vi "Add_Source.vi"(5 "project":refnum<vi>, 7 "IB_Destination.lvclass":refnum<class "IB_Destination.lvclass">, 8 "error in (no error)":errorcluster, 9 "project items":refnum<class "IB_Tree_Item_Proj.lvclass">[](array[class]), 10 "source in":refnum<class "IB_Source.lvclass">[](array[class]), 11 "IB_DestTree in":refnum<class "IB_Tree_Dest.lvclass">) -> (0 "error out":errorcluster, 1 "updated project items":refnum<class "IB_Tree_Item_Proj.lvclass">[](array[class]), 2 "source out":refnum<class "IB_Source.lvclass">[](array[class]), 3 "IB_DestTree out":refnum<class "IB_Tree_Dest.lvclass">)   [LabVIEW 2020, in "IB_Tree_Dest.lvclass"]
uses:
  <vilib>/AppBuilder/IB_Classes/Tree_Dest/IB_Tree_Dest.lvclass
  <vilib>/AppBuilder/IB_Classes/Tree_Dest/IB_Tree_Dest.lvclass/IB_Tree_Dest.ctl
  <vilib>/AppBuilder/IB_Classes/Source/IB_Source.lvclass
  <vilib>/AppBuilder/IB_Classes/Tree/IB_Tree.lvclass
  <vilib>/AppBuilder/IB_Classes/Tree_Item_Proj/IB_Tree_Item_Proj.lvclass
  <vilib>/AppBuilder/IB_Classes/Destination/IB_Destination.lvclass
  <vilib>/AppBuilder/IB_Classes/Tree_Item_Source/IB_Tree_Item_Source.lvclass
  e:/builds/penguin/labview/branches/2020/dev/dist/vi.lib/AppBuilder/IB_Classes/Tree/IB_Tree.lvclass
  e:/builds/penguin/labview/branches/2020/dev/dist/vi.lib/AppBuilder/IB_Classes/Tree_Dest/IB_Tree_Dest.lvclass
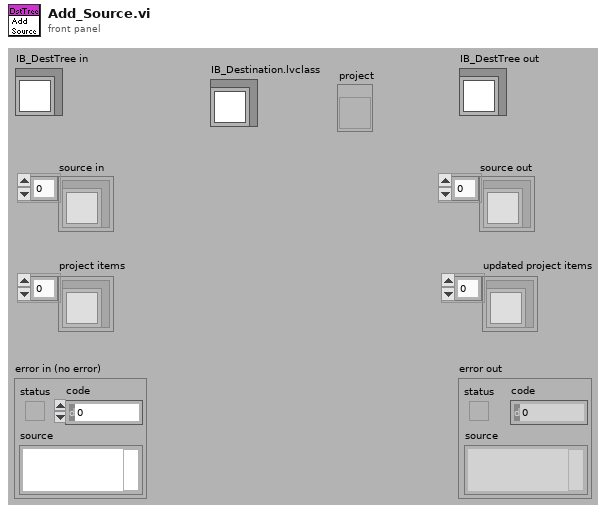
[diagram p1: front panel]
types:
  T1 = typedef "IB_Destination.ctl" = cluster{"name":string, "unlock":bool, "parentTag":string, "destTag":string, "eng_installPath":string}
  T2 = typedef "IB_Tree_Item_Proj.ctl" = cluster{"itemID":string, "path":path}
  T3 = typedef "IB_Source.ctl" = cluster{"name":string, "sourceTag":string, "destTag":string, "path":path, "eng_installPath":string, "UI_inBuild?":bool, "str ref?":bool}
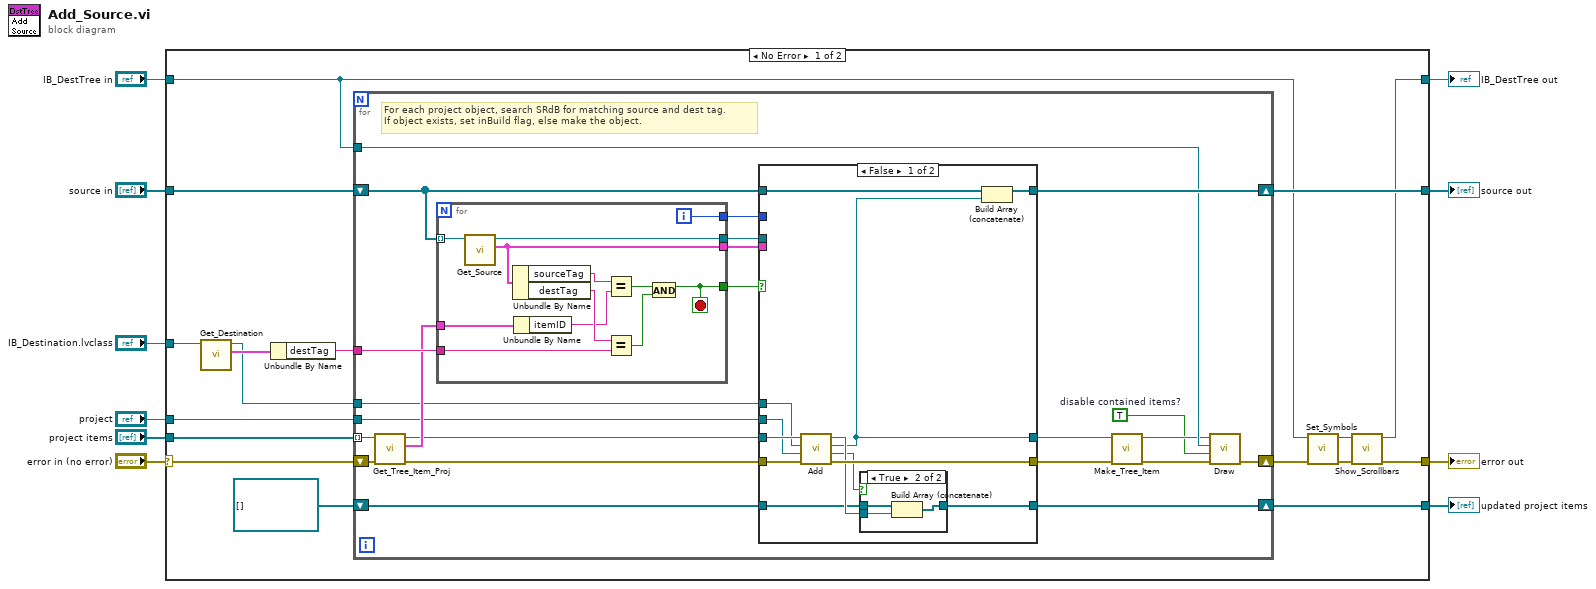
[diagram p0: block diagram]
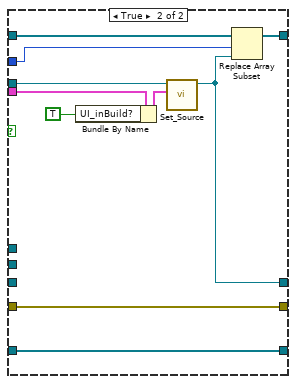
[diagram p3: hidden frame]
diagram:
  n1 = case shown="No Error" "error in (no error)" {
    selector: "error in (no error)" -> [w16 w91]
    tunnel: [w17 w91] -> w9
    tunnel: [w19 w90] -> w7
    tunnel: "IB_DestTree in" -> [w24 w90]
    tunnel: "source in" -> [w27 w89]
    tunnel: "project items" -> [w26 _]
    tunnel: [w25 w89] -> w4
    tunnel: "IB_Destination.lvclass" -> [w14 _]
    tunnel: "project" -> [w15 _]
    tunnel: [w11 _] -> w1
    frame No Error {
      n2 = call <vilib>:"Get_Destination.vi"("IB_Destination in"=w14) -> ("data"=w22:T1, "IB_Destination out"=w13:refnum<class "IB_Destination.lvclass">)  [unwired: 1 in, 8 out]
      n3 = Unbundle By Name(w22) -> ("destTag"=w21:string)
      n4 = for {
        tunnel: w26 -> [w41] mode=indexing
        shift-right: [w49] -> w25
        shift-left: w27 -> [w50]
        tunnel: w24 -> [w36]
        shift-right: [w34] -> w23
        shift-left: w16 -> [w40]
        tunnel: w21 -> [w48]
        tunnel: w13 -> [w38]
        tunnel: w15 -> [w31]
        shift-right: [w29] -> w11
        shift-left: refnum<class "IB_Tree_Item_Proj.lvclass">[] [] ("updated project items") -> [w30]
        w28 = TRUE  # disable contained items?
        # "For each project object, search SRdB for matching source and dest tag.\nIf object exists, set inBuild flag, else make the object."
        n5 = call <vilib>:"Get_Tree_Item_Proj.vi"("error in (no error)"=w40, "IB_TreeProjectItem in"=w41) -> ("error out"=w42:errorcluster, "data"=w44:T2, "IB_TreeProjectItem out"=w43:refnum<class "IB_Tree_Item_Proj.lvclass">)  [unwired: 7 out]
        n6 = for {
          tunnel: w50 -> [w88] mode=indexing
          tunnel: [w86] -> w46
          tunnel: [w81] -> w47
          tunnel: [w85] -> w45
          tunnel: w44 -> [w80]
          tunnel: w48 -> [w78]
          tunnel: [w77] -> w39
          i -> [w85]
          stop <- w81 stop-if-true
          n7 = call <vilib>:"Get_Source.vi"("IB_Source in"=w88) -> ("data"=w77:T3, "IB_Source out"=w86:refnum<class "IB_Source.lvclass">)  [unwired: 1 in, 8 out]
          n8 = Unbundle By Name(w77) -> ("sourceTag"=w87:string, "destTag"=w84:string)
          n9 = Unbundle By Name(w80) -> ("itemID"=w79:string)
          n10 = Equal?(x=w87, y=w79) -> (x = y?=w82:bool)
          n11 = Equal?(x=w84, y=w78) -> (x = y?=w83:bool)
          n12 = And(x=w82, y=w83) -> (x .and. y?=w81:bool)
        }
        n13 = case shown="False" w47 {
          tunnel: w46 -> [_ w69]
          tunnel: w50 -> [w62 w74]
          tunnel: w45 -> [_ w72]
          tunnel: [w61 w73] -> w49
          tunnel: [w57 w71] -> w33
          tunnel: w42 -> [w59 w71]
          tunnel: w43 -> [w60 _]
          tunnel: w39 -> [_ w70]
          tunnel: w38 -> [w58 _]
          tunnel: [w52 w68] -> w37
          tunnel: w31 -> [w56 _]
          tunnel: [w53 w67] -> w29
          tunnel: w30 -> [w54 w67]
          frame False {
            n14 = call-dynamic "Add.vi"("error in (no error)"=w59, "Project"=w56, "IB_Destination.lvclass"=w58, "IB_Tree_Item_Proj in"=w60) -> ("error out"=w57:errorcluster, "updated?"=w51:bool, "IB_Source.lvclass"=w52:refnum<class "IB_Source.lvclass">, "IB_Tree_Item_Proj out"=w55:refnum<class "IB_Tree_Item_Proj.lvclass">)  [unwired: 4 out]
            n15 = case shown="True" w51 {
              tunnel: w54 -> [w63 w66]
              tunnel: w55 -> [_ w65]
              tunnel: [w63 w64] -> w53
              frame False {
              }
              frame True {
                n16 = Build Array (concatenate)(w66, w65) -> (w64:refnum<class "IB_Tree_Item_Proj.lvclass">[])
              }
            }
            n17 = Build Array (concatenate)(w62, w52) -> (w61:refnum<class "IB_Source.lvclass">[])
          }
          frame True {
            n18 = Bundle By Name(cluster=w70, "UI_inBuild?"=TRUE) -> (w76:T3)
            n19 = call <vilib>:"Set_Source.vi"("data"=w76, "IB_Source in"=w69) -> ("IB_Source out"=w68:refnum<class "IB_Source.lvclass">)  [unwired: 1 in, 8 out]
            n20 = Replace Array Subset(array=w74, new element=w68, index=w72) -> (w73:refnum<class "IB_Source.lvclass">[])
          }
        }
        n21 = call-dynamic "Make_Tree_Item.vi"("error in (no error)"=w33, "IB_Source in"=w37) -> ("error out"=w35:errorcluster, "TreeSrcItem"=w32:refnum<class "IB_Tree_Item_Source.lvclass">)  [unwired: 8 out]
        n22 = call-dynamic "Draw.vi"("error in (no error)"=w35, "disable contained items?"=w28, "IB_Tree"=w36, "IB_TreeItem in"=w32) -> ("error out"=w34:errorcluster)  [unwired: 7 out]
      }
      n23 = call <vilib>:"Set_Symbols.vi"("error in (no error)"=w23, "IB_Tree in"=w24) -> ("error out"=w18:errorcluster, "IB_Tree out"=w20:refnum<class "IB_Tree_Dest.lvclass">)  [unwired: 8 out]
      n24 = call <vilib>:"Show_Scrollbars.vi"("error in (no error)"=w18, "IB_Tree in"=w20) -> ("error out"=w17:errorcluster, "IB_Tree out"=w19:refnum<class "IB_Tree_Dest.lvclass">)  [unwired: 8 out]
    }
    frame Error {
    }
  }
  "error out" <- w9
  "IB_DestTree out" <- w7
  "source out" <- w4
  "updated project items" <- w1
